vi "String tokens to string array.vi"(8 "error in (no error)":errorcluster, 11 "String line with tokens":string) -> (0 "error out":errorcluster, 3 "Tokens":string[](array[string]))   [LabVIEW 2013]
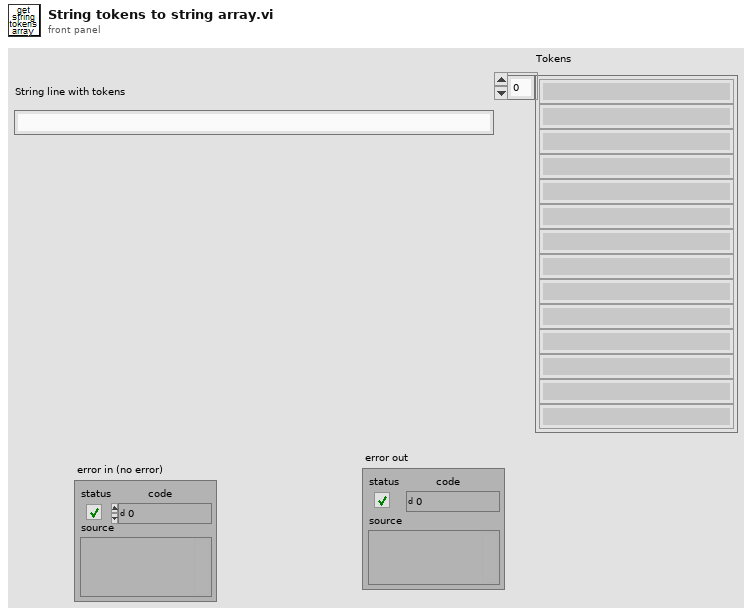
[diagram p1: front panel]
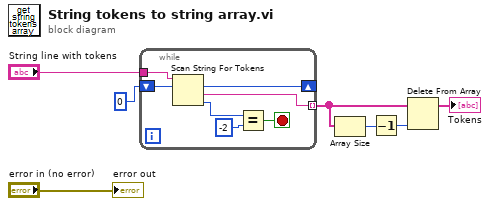
[diagram p0: block diagram]
diagram:
  n1 = while {
    tunnel: "String line with tokens" -> [w14]
    shift-right: [w11] -> _
    shift-left: 0 -> [w13]
    tunnel: [w12] -> w3 mode=indexing
    stop <- w8 stop-if-true
    n2 = Scan String For Tokens(8:w13, 9:w14) -> (0:w10:i32, 1:w12:string, 2:w11:i32)  [unwired: 4 in, 1 out]
    n3 = Equal?(x=w10, y=-2) -> (x = y?=w8:bool)
  }
  n4 = Array Size(array=w3) -> (size(s)=w2:i32)
  n5 = Decrement(x=w2) -> (x-1=w1:i32)
  n6 = Delete From Array(array=w3, index=w1) -> (array with subset deleted=→"Tokens":string[])  [unwired: 1 in, 1 out]
  "error out" <- "error in (no error)"
